vi "Untitled 6 (SubVI).vi"(11 "ConnectionRefIn in":T1) -> (3 "ConnectionRefIn out":T1)   [LabVIEW 2012, in "MBUS_Modbus.lvlib"]
uses:
  MBUS_Modbus.lvlib
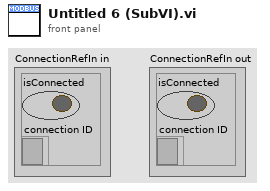
[diagram p1: front panel]
types:
  T1 = cluster{"isConnected":bool, "connection ID":refnum<k5>}
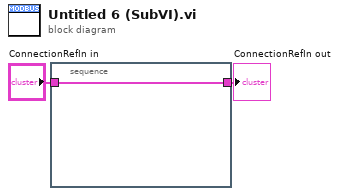
[diagram p0: block diagram]
diagram:
  n1 = stacked-sequence {
    tunnel: "ConnectionRefIn in" -> [w3]
    tunnel: [w3] -> w2
    frame #0 {
    }
  }
  "ConnectionRefIn out" <- w2
